vi "WSVCAP SHL Host LL RFFE Set Configuration Parameters.vi"(0 "RFFE_Clock Divider":u32=20, 5 "RFFE_Slave Address":u8=20, 11 "error in (no error)":errorcluster) -> (15 "error out":errorcluster)   [LabVIEW 2012]
uses:
  Type Defs/WSVCAP SHL Top Level Control Enum.ctl
  Type Defs/WSVCAP SHL Top Level Control Operation Enum.ctl
  Type Defs/WSVCAP SHL State.ctl
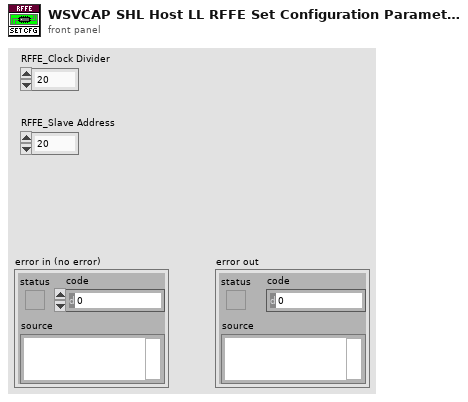
[diagram p1: front panel]
types:
  T1 = typedef "WSVCAP SHL State.ctl" = enum8{"Idle", "Configure I2C", "Configure SPI", "Configure RFFE", "Transfer Data"}
  T2 = typedef "WSVCAP SHL Top Level Control Operation Enum.ctl" = enum16{"Initialize", "Set Control", "Read Control", "Close"}
  T3 = typedef "WSVCAP SHL Top Level Control Enum.ctl" = enum16{"Start", "Cmd", "Transaction", "Wait Ticks", "Socket Mask", "Slave Address", "Sub Address", "Bytes to Write", "Bytes to Read", "Write Data", "Write Flag", "Read Data", "Read Flag", "Ack Read", "Read Status Flag", "Ack Read Status", "Status", "Cycle Count", "Stop Cycle", "Exit"}
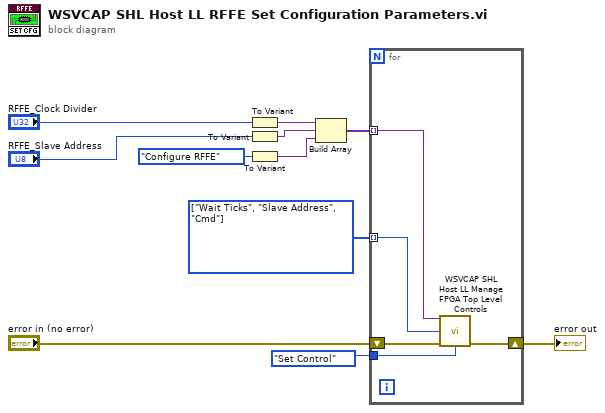
[diagram p0: block diagram]
diagram:
  w6 = T3[] [enum."Wait Ticks", enum."Slave Address", enum."Cmd"] items=["Start", "Cmd", "Transaction", "Wait Ticks", "Socket Mask", "Slave Address", "Sub Address", "Bytes to Write", "Bytes to Read", "Write Data", "Write Flag", "Read Data", "Read Flag", "Ack Read", "Read Status Flag", "Ack Read Status", "Status", "Cycle Count", "Stop Cycle", "Exit"]
  n1 = To Variant(anything="RFFE_Clock Divider") -> (Variant=w9:variant)
  n2 = To Variant(anything="RFFE_Slave Address") -> (Variant=w2:variant)
  n3 = To Variant(anything=WSVCAP_SHL_State."Configure RFFE" ("SPI_Cmd")) -> (Variant=w8:variant)
  n4 = Build Array(w9, w2, w8) -> (w7:variant[])
  n5 = for {
    tunnel: WSVCAP_SHL_Top_Level_Control_Operation_Enum."Set Control" ("Operation") -> [w16]
    tunnel: w7 -> [w15] mode=indexing
    tunnel: w6 -> [w14] mode=indexing
    shift-right: [w12] -> w4
    shift-left: "error in (no error)" -> [w13]
    n6 = call "WSVCAP SHL Host LL Manage FPGA Top Level Controls.vi"("Value In"=w15, "FPGA Top Level Control"=w14, "error in (no error)"=w13, "Operation"=w16) -> ("error out"=w12:errorcluster)  [unwired: 10 in, 1 out]
  }
  "error out" <- w4
